vi "Revert Version.vi"(7 "Index":i32, 8 "error in":errorcluster, 10 "Build Version":T1, 11 "Builder in":refnum<class "Builder.lvclass">) -> (0 "error out":errorcluster, 3 "Builder out":refnum<class "Builder.lvclass">)   [LabVIEW 2021, in "App-Builder Library.lvlib" / "Builder.lvclass"]
uses:
  Builder.lvclass
  <vilib>/AppBuilder/AB_API_Simple/Build Specification Version.ctl
  Builder.lvclass/Builder.ctl
  <vilib>/AppBuilder/AB_API_Simple/Set Build Specification Version (path).vi
  <vilib>/AppBuilder/AB_API_Simple/NI_App_Builder_API.lvlib
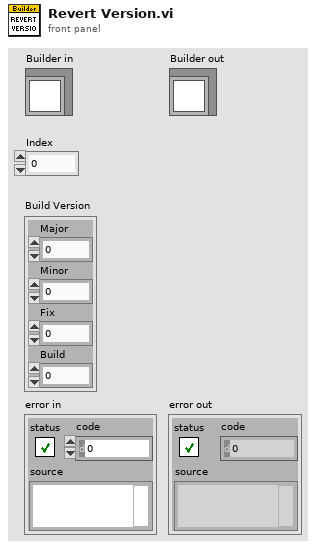
[diagram p1: front panel]
types:
  T1 = typedef "NI_App_Builder_API.lvlib/Build Specification Version.ctl" = cluster{"Major":u16, "Minor":u16, "Fix":u16, "Build":u16}
  T2 = typedef "App-Builder Library.lvlib/Builder.lvclass/Build specification.ctl" = cluster{"target name":string, "Build specification":string, "Project Path":path, "Build Object type":T3}
  T3 = typedef "App-Builder Library.lvlib/Builder.lvclass/Build object type.ctl" = enum16{"EXE", "RT EXE", "Deployable Packed"}
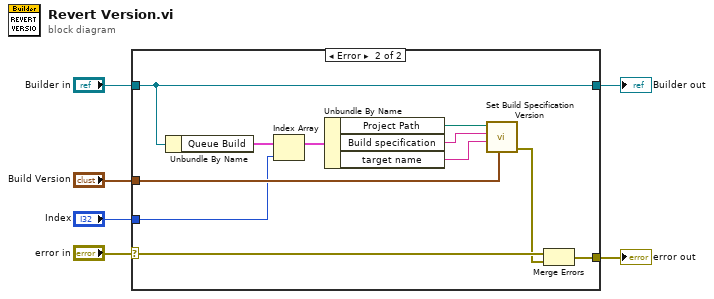
[diagram p0: block diagram]
diagram:
  n1 = case shown="Error" "error in" {
    selector: "error in" -> [w8 w19]
    tunnel: [w8 w16] -> w5
    tunnel: [w7 w17] -> w3
    tunnel: "Builder in" -> [w7 w17]
    tunnel: "Build Version" -> [_ w18]
    tunnel: "Index" -> [_ w9]
    frame No Error {
    }
    frame Error {
      n2 = Unbundle By Name(w17) -> ("Queue Build"=w14:T2[])
      n3 = Index Array(array=w14, index=w9) -> (element=w10:T2)
      n4 = Unbundle By Name(w10) -> ("Project Path"=w13:path, "Build specification"=w11:string, "target name"=w12:string)
      n5 = call-poly <vilib>:"Set Build Specification Version.vi"("Build Specification Version"=w18, "Name of target (My Computer)"=w12, "Name of build specification"=w11, "Path to project"=w13) -> ("error out"=w15:errorcluster)  [unwired: 7 in]
      n6 = Merge Errors(w19, w15) -> (w16:errorcluster)
    }
  }
  "error out" <- w5
  "Builder out" <- w3
